vi "funnels to Commands.vi"(3 "Funnel":T4(array[cluster]), 4 "Funnel Propeties":T2(array[cluster])=[{"Max Speed (um/s)"=2.0, "Direction (For Stroked)"=0, "Orientation (For Filled)"=enum."Vertical", "Curve smooth segments"=20.0, "Bottom Segments"=20.0, "Voltage"=0.0}, {"Max Speed (um/s)"=2.0, "Direction (For Stroked)"=0, "Orientation (For Filled)"=enum."Vertical", "Curve smooth segments"=20.0, "Bottom Segments"=20.0, "Voltage"=0.0}, {"Max Speed (um/s)"=2.0, "Direction (For Stroked)"=0, "Orientation (For Filled)"=enum."Vertical", "Curve smooth segments"=20.0, "Bottom Segments"=20.0, "Voltage"=0.0}, {"Max Speed (um/s)"=2.0, "Direction (For Stroked)"=0, "Orientation (For Filled)"=enum."Vertical", "Curve smooth segments"=20.0, "Bottom Segments"=20.0, "Voltage"=0.0}, {"Max Speed (um/s)"=2.0, "Direction (For Stroked)"=0, "Orientation (For Filled)"=enum."Vertical", "Curve smooth segments"=20.0, "Bottom Segments"=20.0, "Voltage"=0.0}, {"Max Speed (um/s)"=2.0, "Direction (For Stroked)"=0, "Orientation (For Filled)"=enum."Vertical", "Curve smooth segments"=20.0, "Bottom Segments"=20.0, "Voltage"=0.0}, {"Max Speed (um/s)"=2.0, "Direction (For Stroked)"=0, "Orientation (For Filled)"=enum."Vertical", "Curve smooth segments"=20.0, "Bottom Segments"=20.0, "Voltage"=0.0}, {"Max Speed (um/s)"=2.0, "Direction (For Stroked)"=0, "Orientation (For Filled)"=enum."Vertical", "Curve smooth segments"=20.0, "Bottom Segments"=20.0, "Voltage"=0.0}, {"Max Speed (um/s)"=2.0, "Direction (For Stroked)"=0, "Orientation (For Filled)"=enum."Vertical", "Curve smooth segments"=20.0, "Bottom Segments"=20.0, "Voltage"=0.0}, {"Max Speed (um/s)"=2.0, "Direction (For Stroked)"=0, "Orientation (For Filled)"=enum."Vertical", "Curve smooth segments"=20.0, "Bottom Segments"=20.0, "Voltage"=0.0}, {"Max Speed (um/s)"=2.0, "Direction (For Stroked)"=0, "Orientation (For Filled)"=enum."Vertical", "Curve smooth segments"=20.0, "Bottom Segments"=20.0, "Voltage"=0.0}, {"Max Speed (um/s)"=2.0, "Direction (For Stroked)"=0, "Orientation (For Filled)"=enum."Vertical", "Curve smooth segments"=20.0, "Bottom Segments"=20.0, "Voltage"=0.0}, {"Max Speed (um/s)"=2.0, "Direction (For Stroked)"=0, "Orientation (For Filled)"=enum."Vertical", "Curve smooth segments"=20.0, "Bottom Segments"=20.0, "Voltage"=0.0}, {"Max Speed (um/s)"=2.0, "Direction (For Stroked)"=0, "Orientation (For Filled)"=enum."Vertical", "Curve smooth segments"=20.0, "Bottom Segments"=20.0, "Voltage"=0.0}, {"Max Speed (um/s)"=2.0, "Direction (For Stroked)"=0, "Orientation (For Filled)"=enum."Vertical", "Curve smooth segments"=20.0, "Bottom Segments"=20.0, "Voltage"=0.0}, {"Max Speed (um/s)"=2.0, "Direction (For Stroked)"=0, "Orientation (For Filled)"=enum."Vertical", "Curve smooth segments"=20.0, "Bottom Segments"=20.0, "Voltage"=0.0}, {"Max Speed (um/s)"=2.0, "Direction (For Stroked)"=0, "Orientation (For Filled)"=enum."Vertical", "Curve smooth segments"=20.0, "Bottom Segments"=20.0, "Voltage"=0.0}, {"Max Speed (um/s)"=2.0, "Direction (For Stroked)"=0, "Orientation (For Filled)"=enum."Vertical", "Curve smooth segments"=20.0, "Bottom Segments"=20.0, "Voltage"=0.0}, {"Max Speed (um/s)"=2.0, "Direction (For Stroked)"=0, "Orientation (For Filled)"=enum."Vertical", "Curve smooth segments"=20.0, "Bottom Segments"=20.0, "Voltage"=0.0}, {"Max Speed (um/s)"=2.0, "Direction (For Stroked)"=0, "Orientation (For Filled)"=enum."Vertical", "Curve smooth segments"=20.0, "Bottom Segments"=20.0, "Voltage"=0.0}, {"Max Speed (um/s)"=2.0, "Direction (For Stroked)"=0, "Orientation (For Filled)"=enum."Vertical", "Curve smooth segments"=20.0, "Bottom Segments"=20.0, "Voltage"=0.0}, {"Max Speed (um/s)"=2.0, "Direction (For Stroked)"=0, "Orientation (For Filled)"=enum."Vertical", "Curve smooth segments"=20.0, "Bottom Segments"=20.0, "Voltage"=0.0}, {"Max Speed (um/s)"=2.0, "Direction (For Stroked)"=0, "Orientation (For Filled)"=enum."Vertical", "Curve smooth segments"=20.0, "Bottom Segments"=20.0, "Voltage"=0.0}, {"Max Speed (um/s)"=2.0, "Direction (For Stroked)"=0, "Orientation (For Filled)"=enum."Vertical", "Curve smooth segments"=20.0, "Bottom Segments"=20.0, "Voltage"=0.0}, {"Max Speed (um/s)"=2.0, "Direction (For Stroked)"=0, "Orientation (For Filled)"=enum."Vertical", "Curve smooth segments"=20.0, "Bottom Segments"=20.0, "Voltage"=0.0}, {"Max Speed (um/s)"=2.0, "Direction (For Stroked)"=0, "Orientation (For Filled)"=enum."Vertical", "Curve smooth segments"=20.0, "Bottom Segments"=20.0, "Voltage"=0.0}, {"Max Speed (um/s)"=2.0, "Direction (For Stroked)"=0, "Orientation (For Filled)"=enum."Vertical", "Curve smooth segments"=20.0, "Bottom Segments"=20.0, "Voltage"=0.0}, {"Max Speed (um/s)"=2.0, "Direction (For Stroked)"=0, "Orientation (For Filled)"=enum."Vertical", "Curve smooth segments"=20.0, "Bottom Segments"=20.0, "Voltage"=0.0}, {"Max Speed (um/s)"=2.0, "Direction (For Stroked)"=0, "Orientation (For Filled)"=enum."Vertical", "Curve smooth segments"=20.0, "Bottom Segments"=20.0, "Voltage"=0.0}, {"Max Speed (um/s)"=2.0, "Direction (For Stroked)"=0, "Orientation (For Filled)"=enum."Vertical", "Curve smooth segments"=20.0, "Bottom Segments"=20.0, "Voltage"=0.0}] {"Direction (For Stroked)" items=["Forward", "Backward"]}) -> (1 "Lithography information":T1(array[cluster]))   [LabVIEW 2013]
doc: "This VI processes the rectangles' data and outputs lithography data."
uses:
  <vilib>/Analysis/Matrix/Datatypes/RealMatrix.ctl
  simulator/Global Variables.vi
  <vilib>/Analysis/Matrix/NI_Matrix.lvlib
panel:
  out "error out":errorcluster
  in  "error in (no error)":errorcluster
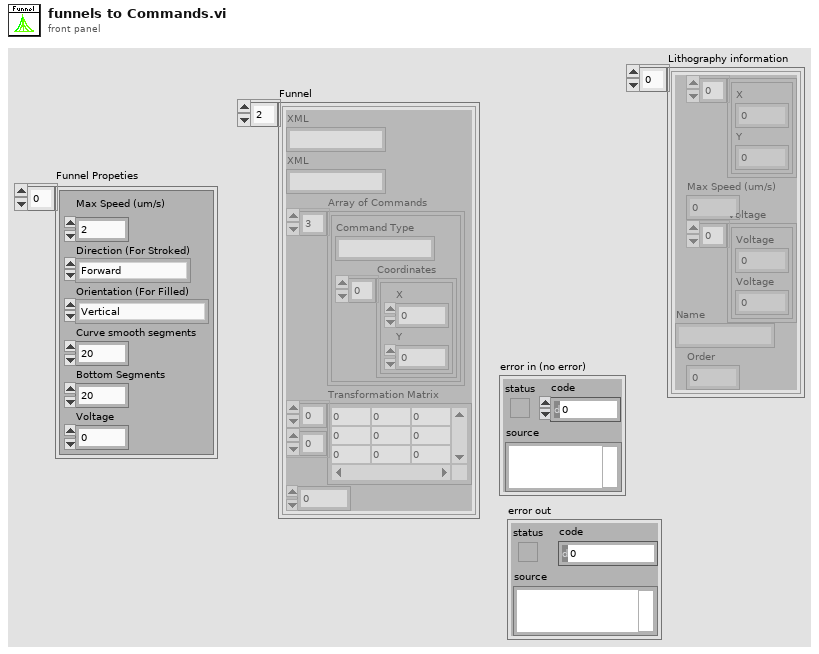
[diagram p1: front panel]
types:
  T1 = cluster{cluster{"X":dbl, "Y":dbl}[], "Max Speed (um/s)":dbl, "Voltage":cluster{"Voltage":dbl, "Voltage":dbl}[], "Name":string, "Order":i32}[]
  T2 = cluster{"Max Speed (um/s)":dbl, "Direction (For Stroked)":u16, "Orientation (For Filled)":enum16{"Horizontal", "Vertical"}, "Curve smooth segments":dbl, "Bottom Segments":dbl, "Voltage":dbl}[]
  T3 = typedef "NI_Matrix.lvlib/RealMatrix.ctl" = dbl[][]
  T4 = cluster{"XML":string, "XML":string, "Array of Commands":cluster{"Command Type":string, "Coordinates":cluster{"X":dbl, "Y":dbl}[]}[], "Transformation Matrix":T3, "Order":i32}[]
  T5 = cluster{"Command Type":string, "Coordinates":cluster{"X":dbl, "Y":dbl}[]}[]
  T6 = cluster{"Command Type":string, "Coordinates":cluster{"X":dbl, "Y":dbl}[]}
  T7 = cluster{cluster{"X":dbl, "Y":dbl}[], "Max Speed (um/s)":dbl, cluster{"Voltage":dbl, "Voltage":dbl}[], string, "Order":i32}
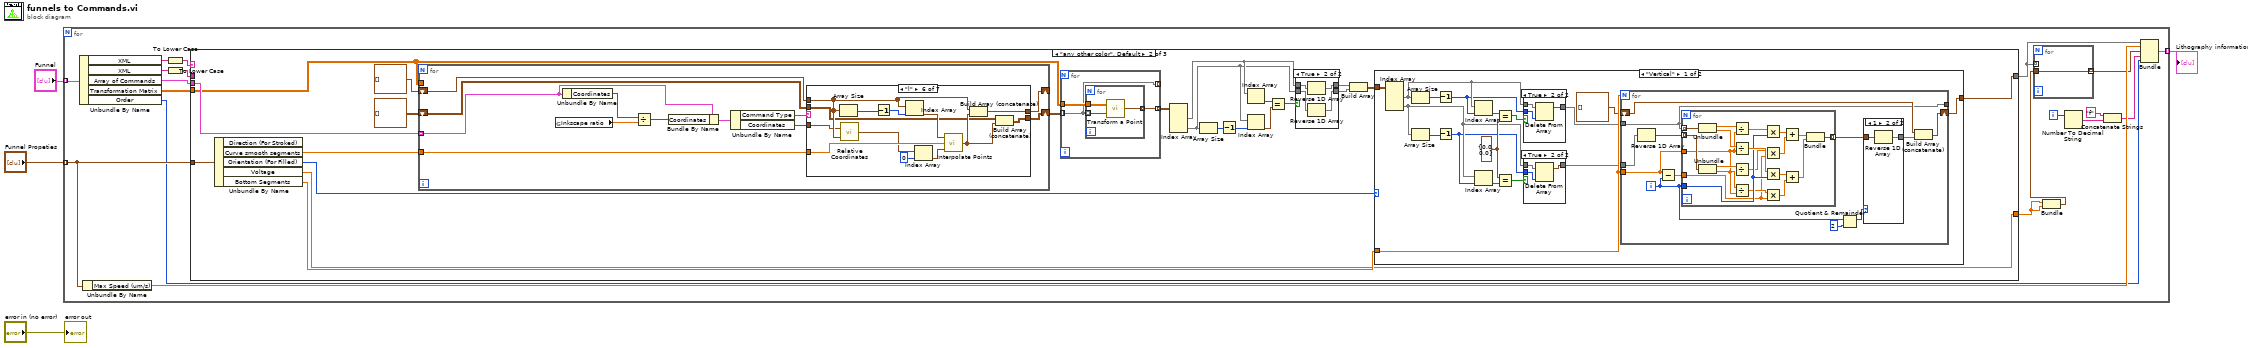
[diagram p0: block diagram]
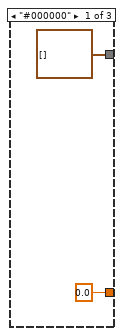
[diagram p2: hidden frame]
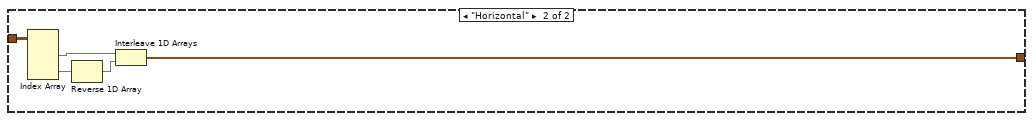
[diagram p7: hidden frame]
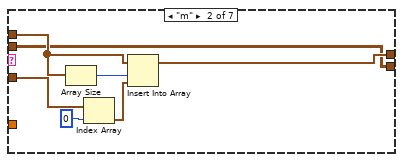
[diagram p9: hidden frame]
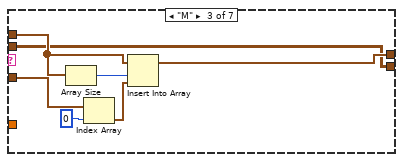
[diagram p10: hidden frame]
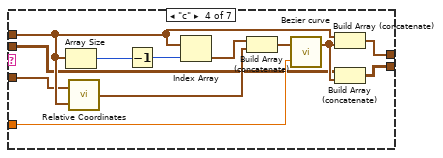
[diagram p11: hidden frame]
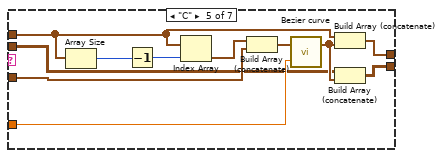
[diagram p12: hidden frame]
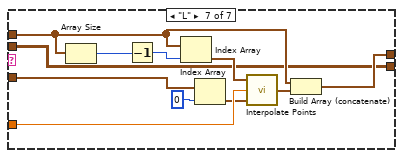
[diagram p13: hidden frame]
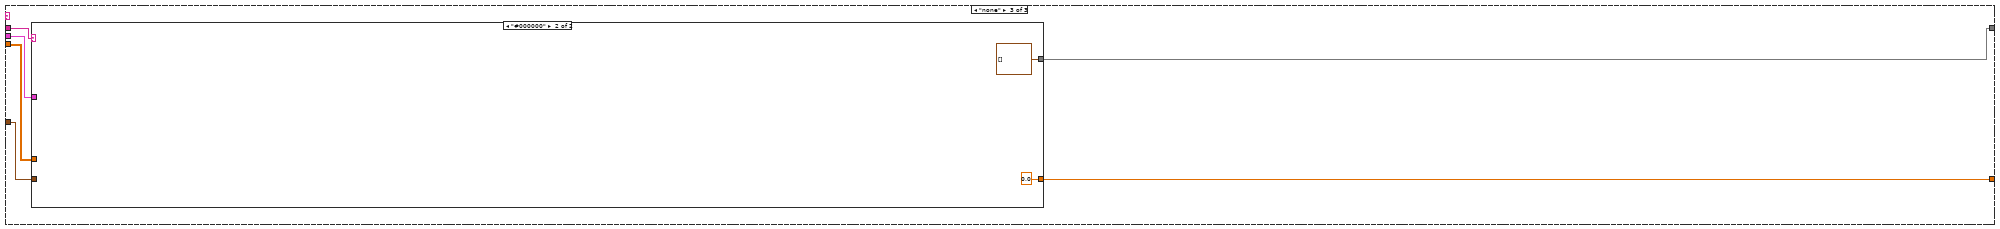
[diagram p14: hidden frame]
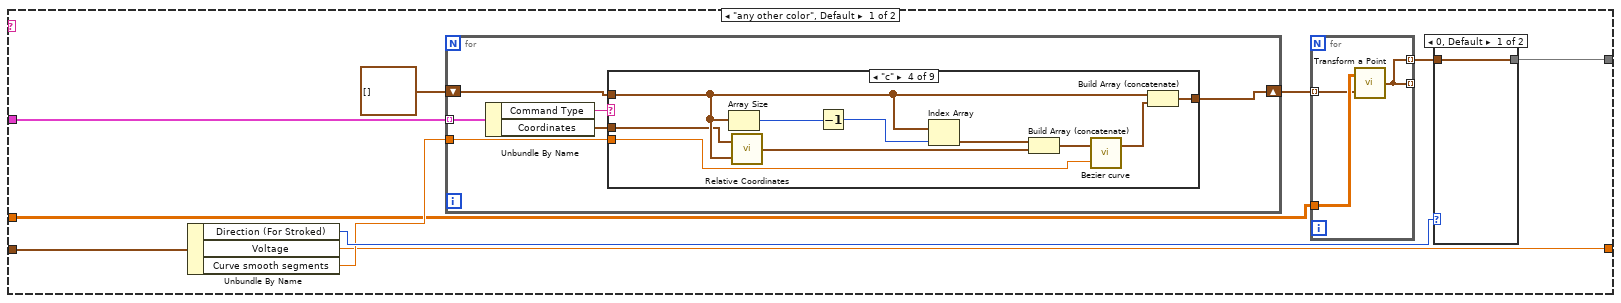
[diagram p15: hidden frame]
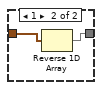
[diagram p16: hidden frame]
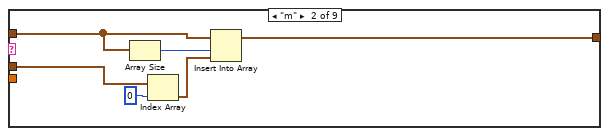
[diagram p18: hidden frame]
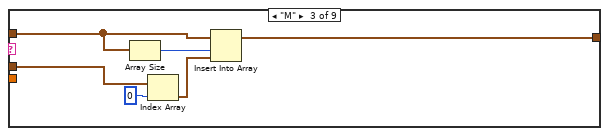
[diagram p19: hidden frame]
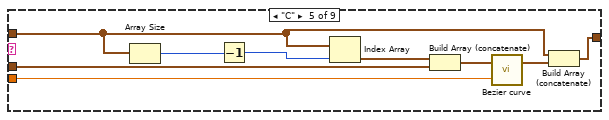
[diagram p20: hidden frame]
diagram:
  n1 = for {
    tunnel: "Funnel" -> [w16] mode=indexing
    tunnel: "Funnel Propeties" -> [w18] mode=indexing
    tunnel: [w19] -> w1 mode=indexing
    i -> [w11]
    n2 = Unbundle By Name(w16) -> ("XML"=w23:string, "XML"=w21:string, "Array of Commands"=w15:T5, "Transformation Matrix"=w10:T3, "Order"=w9:i32)
    n3 = Unbundle By Name(w18) -> ("Max Speed (um/s)"=w17:dbl)
    n4 = To Lower Case(string=w23) -> (all lower case string=w22:string)
    n5 = To Lower Case(string=w21) -> (all lower case string=w20:string)
    n6 = case shown="\"any other color\", Default" w22 {
      tunnel: w20 -> [_ _ w202]
      tunnel: w18 -> [_ w47 w205]
      tunnel: [cluster{"X":dbl, "Y":dbl}[] [] w42 w204] -> w8
      tunnel: w15 -> [_ w46 w206]
      tunnel: w10 -> [_ w40 w203]
      tunnel: [0.0 ("Voltage") w27 w201] -> w6
      frame "#000000" {
      }
      frame "any other color", Default {
        n7 = Unbundle By Name(w47) -> ("Curve smooth segments"=w43:dbl, "Orientation (For Filled)"=w44:enum16{"Horizontal", "Vertical"}, "Voltage"=w27:dbl, "Bottom Segments"=w41:dbl)  [unwired: 1 out]
        n8 = for {
          tunnel: w46 -> [w127] mode=indexing
          shift-right: [w134] -> _
          shift-left: cluster{"X":dbl, "Y":dbl}[] [] -> [w136]
          tunnel: w43 -> [w135]
          tunnel: w40 -> [_]
          shift-right: [w132] -> w39
          shift-left: cluster{"X":dbl, "Y":dbl}[][] [] -> [w131]
          n9 = global read "Global Variables.vi" "Inkscape ratio"() -> (w129:dbl)
          n10 = Unbundle By Name(w127) -> ("Coordinates"=w130:cluster{"X":dbl, "Y":dbl}[])
          n11 = Divide(x=w130, y=w129) -> (x/y=w128:cluster{"X":dbl, "Y":dbl}[])
          n12 = Bundle By Name(cluster=w127, "Coordinates"=w128) -> (w126:T6)
          n13 = Unbundle By Name(w126) -> ("Command Type"=w137:string, "Coordinates"=w133:cluster{"X":dbl, "Y":dbl}[])
          n14 = case shown="\"l\"" w137 {
            tunnel: w133 -> [_ w141 w148 w157 w169 w180 w197]
            tunnel: w136 -> [w139 w143 w149 w165 w176 w182 w198]
            tunnel: [w139 w144 w150 w159 w171 w188 w199] -> w134
            tunnel: w135 -> [_ _ _ w158 w170 w189 w200]
            tunnel: [w138 w140 w147 w156 w167 w178 w190] -> w132
            tunnel: w131 -> [w138 w140 w147 w154 w166 w177 w190]
            frame "other letters", Default {
            }
            frame "m" {
              n15 = Array Size(array=w143) -> (size(s)=w146:i32)
              n16 = Index Array(array=w141, index=0) -> (element=w145:cluster{"X":dbl, "Y":dbl})
              n17 = Insert Into Array(array=w143, index=w146, new element=w145) -> (w144:cluster{"X":dbl, "Y":dbl}[])
            }
            frame "M" {
              n18 = Array Size(array=w149) -> (size(s)=w152:i32)
              n19 = Index Array(array=w148, index=0) -> (element=w151:cluster{"X":dbl, "Y":dbl})
              n20 = Insert Into Array(array=w149, index=w152, new element=w151) -> (w150:cluster{"X":dbl, "Y":dbl}[])
            }
            frame "c" {
              n21 = Array Size(array=w165) -> (size(s)=w161:i32)
              n22 = call "Relative Coordinates.vi"("All Coordinates"=w165, "Command Coordinates"=w157) -> ("Adjusted Command Coordinates"=w163:cluster{"X":dbl, "Y":dbl}[])
              n23 = Decrement(x=w161) -> (x-1=w160:i32)
              n24 = Index Array(array=w165, index=w160) -> (element=w164:cluster{"X":dbl, "Y":dbl})
              n25 = Build Array (concatenate)(w164, w163) -> (w162:cluster{"X":dbl, "Y":dbl}[])
              n26 = call "Bezier curve.vi"("Segments"=w158, "Parameters"=w162) -> ("Coordinate Array"=w155:cluster{"X":dbl, "Y":dbl}[])  [unwired: 1 out]
              n27 = Build Array (concatenate)(w165, w155) -> (w159:cluster{"X":dbl, "Y":dbl}[])
              n28 = Build Array (concatenate)(w154, w155) -> (w156:cluster{"X":dbl, "Y":dbl}[][])
            }
            frame "C" {
              n29 = Array Size(array=w176) -> (size(s)=w173:i32)
              n30 = Decrement(x=w173) -> (x-1=w172:i32)
              n31 = Index Array(array=w176, index=w172) -> (element=w175:cluster{"X":dbl, "Y":dbl})
              n32 = Build Array (concatenate)(w175, w169) -> (w174:cluster{"X":dbl, "Y":dbl}[])
              n33 = call "Bezier curve.vi"("Segments"=w170, "Parameters"=w174) -> ("Coordinate Array"=w168:cluster{"X":dbl, "Y":dbl}[])  [unwired: 1 out]
              n34 = Build Array (concatenate)(w176, w168) -> (w171:cluster{"X":dbl, "Y":dbl}[])
              n35 = Build Array (concatenate)(w166, w168) -> (w167:cluster{"X":dbl, "Y":dbl}[][])
            }
            frame "l" {
              n36 = Array Size(array=w182) -> (size(s)=w184:i32)
              n37 = call "Relative Coordinates.vi"("All Coordinates"=w182, "Command Coordinates"=w180) -> ("Adjusted Command Coordinates"=w187:cluster{"X":dbl, "Y":dbl}[])
              n38 = Decrement(x=w184) -> (x-1=w183:i32)
              n39 = Index Array(array=w182, index=w183) -> (element=w186:cluster{"X":dbl, "Y":dbl})
              n40 = Index Array(array=w187, index=0) -> (element=w185:cluster{"X":dbl, "Y":dbl})
              n41 = call "Interpolate Points.vi"("End Point"=w185, "Distance between Points"=w189, "Start Point"=w186) -> ("Output Point Array"=w179:cluster{"X":dbl, "Y":dbl}[])
              n42 = Build Array (concatenate)(w182, w179) -> (w188:cluster{"X":dbl, "Y":dbl}[])
              n43 = Build Array (concatenate)(w177, w179) -> (w178:cluster{"X":dbl, "Y":dbl}[][])
            }
            frame "L" {
              n44 = Array Size(array=w198) -> (size(s)=w193:i32)
              n45 = Decrement(x=w193) -> (x-1=w192:i32)
              n46 = Index Array(array=w198, index=w192) -> (element=w196:cluster{"X":dbl, "Y":dbl})
              n47 = Index Array(array=w197, index=0) -> (element=w194:cluster{"X":dbl, "Y":dbl})
              n48 = call "Interpolate Points.vi"("End Point"=w194, "Distance between Points"=w200, "Start Point"=w196) -> ("Output Point Array"=w191:cluster{"X":dbl, "Y":dbl}[])
              n49 = Build Array (concatenate)(w198, w191) -> (w199:cluster{"X":dbl, "Y":dbl}[])
            }
          }
        }
        n50 = for {
          tunnel: [w56] -> w38 mode=indexing
          tunnel: w40 -> [w57]
          tunnel: [w55] -> _ mode=indexing
          tunnel: w39 -> [w55] mode=indexing
          n51 = for {
            tunnel: w57 -> [w60]
            tunnel: [w59] -> w56 mode=indexing
            tunnel: w55 -> [w58] mode=indexing
            n52 = call "Transform a Point.vi"("Point to Transform"=w58, "Transformation Matrix"=w60) -> ("Transformed Point"=w59:cluster{"X":dbl, "Y":dbl})
          }
        }
        n53 = Index Array(array=w38) -> (element #1=w31:cluster{"X":dbl, "Y":dbl}[], element #2=w30:cluster{"X":dbl, "Y":dbl}[])  [unwired: 4 in]
        n54 = Array Size(array=w30) -> (size(s)=w36:i32)
        n55 = Decrement(x=w36) -> (x-1=w35:i32)
        n56 = Index Array(array=w31) -> (element=w34:cluster{"X":dbl, "Y":dbl})  [unwired: 1 in]
        n57 = Index Array(array=w30, index=w35) -> (element=w33:cluster{"X":dbl, "Y":dbl})
        n58 = Equal?(x=w34, y=w33) -> (x = y?=w32:bool)
        n59 = case shown="True" w32 {
          tunnel: w31 -> [w50 w54]
          tunnel: w30 -> [w49 w53]
          tunnel: [w50 w52] -> w29
          tunnel: [w49 w51] -> w28
          frame False {
          }
          frame True {
            n60 = Reverse 1D Array(array=w54) -> (reversed array=w52:cluster{"X":dbl, "Y":dbl}[])
            n61 = Reverse 1D Array(array=w53) -> (reversed array=w51:cluster{"X":dbl, "Y":dbl}[])
          }
        }
        n62 = Build Array(w29, w28) -> (w37:cluster{"X":dbl, "Y":dbl}[][])
        n63 = case shown="\"Vertical\"" w44 {
          tunnel: w37 -> [w77 w125]
          tunnel: [w76 w121] -> w42
          tunnel: w41 -> [w75 _]
          frame "Vertical" {
            w71 = cluster{"X":dbl, "Y":dbl} {"X"=0.0, "Y"=0.0} ("y")
            n64 = Index Array(array=w77) -> (element #1=w68:cluster{"X":dbl, "Y":dbl}[], element #2=w64:cluster{"X":dbl, "Y":dbl}[])  [unwired: 4 in]
            n65 = Array Size(array=w68) -> (size(s)=w69:i32)
            n66 = Array Size(array=w64) -> (size(s)=w70:i32)
            n67 = Decrement(x=w69) -> (x-1=w67:i32)
            n68 = Decrement(x=w70) -> (x-1=w63:i32)
            n69 = Index Array(array=w68, index=w67) -> (element=w73:cluster{"X":dbl, "Y":dbl})
            n70 = Index Array(array=w64, index=w63) -> (element=w72:cluster{"X":dbl, "Y":dbl})
            n71 = Equal?(x=w73, y=w71) -> (x = y?=w65:bool)
            n72 = Equal?(x=w71, y=w72) -> (x = y?=w61:bool)
            n73 = case shown="True" w65 {
              tunnel: w68 -> [w82 w85]
              tunnel: w67 -> [_ w83]
              tunnel: [w82 w84] -> w66
              frame False {
              }
              frame True {
                n74 = Delete From Array(array=w85, index=w83) -> (array with subset deleted=w84:cluster{"X":dbl, "Y":dbl}[])  [unwired: 1 in, 1 out]
              }
            }
            n75 = case shown="True" w61 {
              tunnel: w64 -> [w78 w81]
              tunnel: w63 -> [_ w79]
              tunnel: [w78 w80] -> w62
              frame False {
              }
              frame True {
                n76 = Delete From Array(array=w81, index=w79) -> (array with subset deleted=w80:cluster{"X":dbl, "Y":dbl}[])  [unwired: 1 in, 1 out]
              }
            }
            n77 = for {
              N: w75 -> [_]
              tunnel: [w86] -> _
              tunnel: w62 -> [w87]
              tunnel: w75 -> [w94]
              shift-right: [w96] -> w76
              shift-left: cluster{dbl, dbl}[] [] -> [w95]
              tunnel: w66 -> [w86]
              i -> [w92]
              n78 = Reverse 1D Array(array=w87) -> (reversed array=w93:cluster{"X":dbl, "Y":dbl}[])
              n79 = Subtract(x=w94, y=w92) -> (x-y=w97:dbl)
              n80 = for {
                tunnel: w86 -> [w120] mode=indexing
                tunnel: w93 -> [w119] mode=indexing
                tunnel: w94 -> [w111]
                tunnel: w92 -> [w114]
                tunnel: w97 -> [w108]
                tunnel: [w101] -> w89 mode=indexing
                n81 = Unbundle(w120) -> ("X"=w118:dbl, "Y"=w116:dbl)
                n82 = Unbundle(w119) -> ("X"=w113:dbl, "Y"=w112:dbl)
                n83 = Divide(x=w118, y=w111) -> (x/y=w117:dbl)
                n84 = Divide(x=w116, y=w111) -> (x/y=w115:dbl)
                n85 = Divide(x=w113, y=w111) -> (x/y=w110:dbl)
                n86 = Divide(x=w112, y=w111) -> (x/y=w109:dbl)
                n87 = Multiply(x=w117, y=w114) -> (x*y=w106:dbl)
                n88 = Multiply(x=w110, y=w108) -> (x*y=w105:dbl)
                n89 = Multiply(x=w115, y=w114) -> (x*y=w104:dbl)
                n90 = Multiply(x=w109, y=w108) -> (x*y=w103:dbl)
                n91 = Add(x=w106, y=w105) -> (x+y=w102:dbl)
                n92 = Add(x=w104, y=w103) -> (x+y=w107:dbl)
                n93 = Bundle(w102, w107) -> (w101:cluster{dbl, dbl})  [unwired: 1 in]
              }
              n94 = Quotient & Remainder(x=w92, y=2) -> (x-y*floor(x/y)=w90:i32)  [unwired: 1 out]
              n95 = case shown="1" w90 {
                tunnel: w89 -> [w98 w100]
                tunnel: [w98 w99] -> w88
                frame 0, Default {
                }
                frame 1 {
                  n96 = Reverse 1D Array(array=w100) -> (reversed array=w99:cluster{dbl, dbl}[])
                }
              }
              n97 = Build Array (concatenate)(w95, w88) -> (w96:cluster{dbl, dbl}[])
            }
          }
          frame "Horizontal" {
            n98 = Index Array(array=w125) -> (element #1=w123:cluster{"X":dbl, "Y":dbl}[], element #2=w124:cluster{"X":dbl, "Y":dbl}[])  [unwired: 4 in]
            n99 = Reverse 1D Array(array=w124) -> (reversed array=w122:cluster{"X":dbl, "Y":dbl}[])
            n100 = Interleave 1D Arrays(w123, w122) -> (w121:cluster{"X":dbl, "Y":dbl}[])
          }
        }
      }
      frame "none" {
        n101 = case shown="\"#000000\"" w202 {
          tunnel: w206 -> [w216 _]
          tunnel: w205 -> [w214 _]
          tunnel: [w213 cluster{"X":dbl, "Y":dbl}[] []] -> w204
          tunnel: w203 -> [w210 _]
          tunnel: [w207 0.0 ("Voltage")] -> w201
          frame "any other color", Default {
            n102 = Unbundle By Name(w214) -> ("Direction (For Stroked)"=w212:u16, "Voltage"=w207:dbl, "Curve smooth segments"=w211:dbl)
            n103 = for {
              tunnel: w216 -> [w228] mode=indexing
              shift-right: [w224] -> w209
              shift-left: cluster{"X":dbl, "Y":dbl}[] [] -> [w225]
              tunnel: w211 -> [w223]
              n104 = Unbundle By Name(w228) -> ("Command Type"=w227:string, "Coordinates"=w226:cluster{"X":dbl, "Y":dbl}[])
              n105 = case shown="\"c\"" w227 {
                tunnel: w226 -> [_ w230 w236 w242 w252 w261 w265 _ _]
                tunnel: w225 -> [w229 w231 w237 w249 w258 w263 w267 w268 w273]
                tunnel: [w229 w232 w238 w251 w260 w262 w266 w269 w274] -> w224
                tunnel: w223 -> [_ _ _ w243 w253 _ _ _ _]
                frame "other letters", Default {
                }
                frame "m" {
                  n106 = Array Size(array=w231) -> (size(s)=w234:i32)
                  n107 = Index Array(array=w230, index=0) -> (element=w233:cluster{"X":dbl, "Y":dbl})
                  n108 = Insert Into Array(array=w231, index=w234, new element=w233) -> (w232:cluster{"X":dbl, "Y":dbl}[])
                }
                frame "M" {
                  n109 = Array Size(array=w237) -> (size(s)=w240:i32)
                  n110 = Index Array(array=w236, index=0) -> (element=w239:cluster{"X":dbl, "Y":dbl})
                  n111 = Insert Into Array(array=w237, index=w240, new element=w239) -> (w238:cluster{"X":dbl, "Y":dbl}[])
                }
                frame "c" {
                  n112 = Array Size(array=w249) -> (size(s)=w245:i32)
                  n113 = call "Relative Coordinates.vi"("All Coordinates"=w249, "Command Coordinates"=w242) -> ("Adjusted Command Coordinates"=w247:cluster{"X":dbl, "Y":dbl}[])
                  n114 = Decrement(x=w245) -> (x-1=w244:i32)
                  n115 = Index Array(array=w249, index=w244) -> (element=w248:cluster{"X":dbl, "Y":dbl})
                  n116 = Build Array (concatenate)(w248, w247) -> (w246:cluster{"X":dbl, "Y":dbl}[])
                  n117 = call "Bezier curve.vi"("Segments"=w243, "Parameters"=w246) -> ("Coordinate Array"=w250:cluster{"X":dbl, "Y":dbl}[])  [unwired: 1 out]
                  n118 = Build Array (concatenate)(w249, w250) -> (w251:cluster{"X":dbl, "Y":dbl}[])
                }
                frame "C" {
                  n119 = Array Size(array=w258) -> (size(s)=w255:i32)
                  n120 = Decrement(x=w255) -> (x-1=w254:i32)
                  n121 = Index Array(array=w258, index=w254) -> (element=w257:cluster{"X":dbl, "Y":dbl})
                  n122 = Build Array (concatenate)(w257, w252) -> (w256:cluster{"X":dbl, "Y":dbl}[])
                  n123 = call "Bezier curve.vi"("Segments"=w253, "Parameters"=w256) -> ("Coordinate Array"=w259:cluster{"X":dbl, "Y":dbl}[])  [unwired: 1 out]
                  n124 = Build Array (concatenate)(w258, w259) -> (w260:cluster{"X":dbl, "Y":dbl}[])
                }
                frame "l" {
                  n125 = call "Relative Coordinates.vi"("All Coordinates"=w263, "Command Coordinates"=w261) -> ("Adjusted Command Coordinates"=w264:cluster{"X":dbl, "Y":dbl}[])
                  n126 = Build Array (concatenate)(w263, w264) -> (w262:cluster{"X":dbl, "Y":dbl}[])
                }
                frame "L" {
                  n127 = Build Array (concatenate)(w267, w265) -> (w266:cluster{"X":dbl, "Y":dbl}[])
                }
                frame "z" {
                  n128 = Array Size(array=w268) -> (size(s)=w271:i32)
                  n129 = Index Array(array=w268, index=0) -> (element=w270:cluster{"X":dbl, "Y":dbl})
                  n130 = Insert Into Array(array=w268, index=w271, new element=w270) -> (w269:cluster{"X":dbl, "Y":dbl}[])
                }
                frame "Z" {
                  n131 = Array Size(array=w273) -> (size(s)=w276:i32)
                  n132 = Index Array(array=w273, index=0) -> (element=w275:cluster{"X":dbl, "Y":dbl})
                  n133 = Insert Into Array(array=w273, index=w276, new element=w275) -> (w274:cluster{"X":dbl, "Y":dbl}[])
                }
              }
            }
            n134 = for {
              tunnel: [w217] -> _ mode=indexing
              tunnel: w210 -> [w219]
              tunnel: w209 -> [w218] mode=indexing
              tunnel: [w217] -> w208 mode=indexing
              n135 = call "Transform a Point.vi"("Point to Transform"=w218, "Transformation Matrix"=w219) -> ("Transformed Point"=w217:cluster{"X":dbl, "Y":dbl})
            }
            n136 = case shown="0, Default" w212 {
              tunnel: [w220 w221] -> w213
              tunnel: w208 -> [w220 w222]
              frame 0, Default {
              }
              frame 1 {
                n137 = Reverse 1D Array(array=w222) -> (reversed array=w221:cluster{"X":dbl, "Y":dbl}[])
              }
            }
          }
          frame "#000000" {
          }
        }
      }
    }
    n138 = Bundle("Voltage"=w6, "Voltage"=w6) -> (w5:cluster{"Voltage":dbl, "Voltage":dbl})  [unwired: 1 in]
    n139 = for {
      tunnel: w8 -> [_] mode=indexing
      tunnel: w5 -> [w24]
      tunnel: [w24] -> w7 mode=indexing
    }
    n140 = Number To Decimal String(number=w11) -> (decimal integer string=w13:string)  [unwired: 1 in]
    n141 = Concatenate Strings("f", w13) -> (w12:string)
    n142 = Bundle(w8, "Max Speed (um/s)"=w17, w7, w12, "Order"=w9) -> (w19:T7)  [unwired: 1 in]
  }
  "Lithography information" <- w1
  "error out" <- "error in (no error)"
